vi "ObatainMessage.vi"(8 "error in (no error)":errorcluster, 10 "COM Bluegiga in":refnum<visa-resource-name>, 11 "BLE Message in":refnum<class "BLE Message.lvclass">) -> (0 "error out":errorcluster, 3 "BLE Message out":refnum<class "BLE Message.lvclass">)   [LabVIEW 2015, in "BLE Message.lvclass"]
uses:
  BLE Message.lvclass
  BLE Message.lvclass/BLE Message.ctl
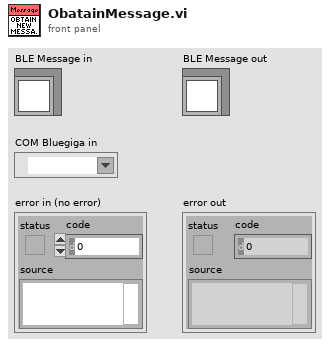
[diagram p1: front panel]
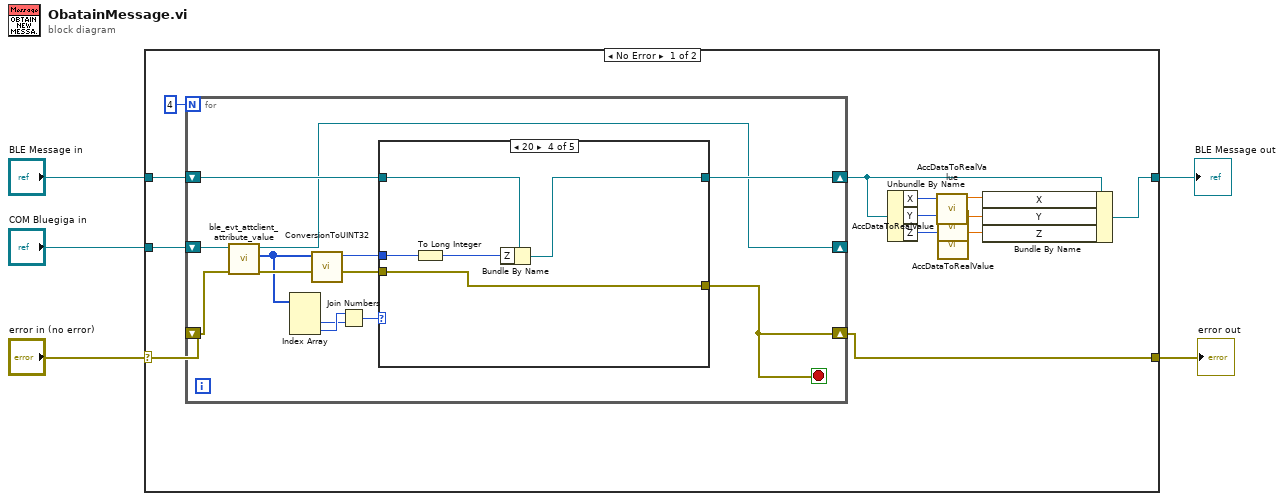
[diagram p0: block diagram]
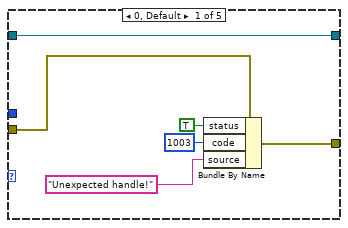
[diagram p2: hidden frame]
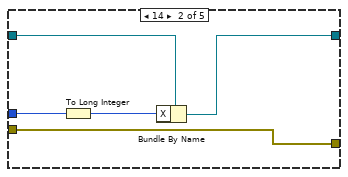
[diagram p3: hidden frame]
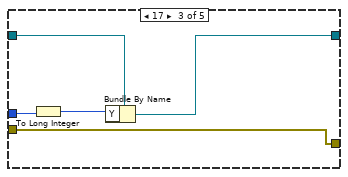
[diagram p4: hidden frame]
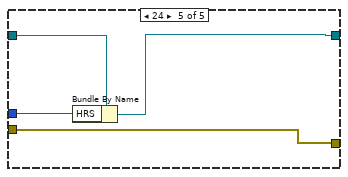
[diagram p5: hidden frame]
diagram:
  n1 = case shown="No Error" "error in (no error)" {
    selector: "error in (no error)" -> [w16 w57]
    tunnel: [w14 w57] -> w4
    tunnel: [w6 w56] -> w2
    tunnel: "BLE Message in" -> [w18 w56]
    tunnel: "COM Bluegiga in" -> [w17 _]
    frame No Error {
      n2 = for {
        N: 4 -> [_]
        shift-right: [w20] -> w14
        shift-left: w16 -> [w29]
        shift-right: [w21] -> w13
        shift-left: w18 -> [w26]
        shift-right: [w19] -> _
        shift-left: w17 -> [w30]
        stop <- w20 stop-if-true
        n3 = call <vilib>:"ble_evt_attclient_attribute_value.vi"("error in (no error)"=w29, "COM Bluegiga in"=w30) -> ("error out"=w24:errorcluster, "characteristic value"=w23:u8[], "COM Bluegiga out"=w19:refnum<visa-resource-name>)  [unwired: 6 in, 1 out]
        n4 = Index Array(array=w23) -> (element #2=w27:u8, element #3=w28:u8)  [unwired: 3 in, 1 out]
        n5 = call "ConversionToUINT32.vi"("uint byte tab"=w23) -> ("Outcome"=w22:u32)  [unwired: 10 in]
        n6 = Join Numbers(hi=w28, lo=w27) -> ((hi.lo)=w25:u16)
        n7 = case shown="20" w25 {
          tunnel: w26 -> [w31 w41 w46 w51 w55]
          tunnel: w24 -> [w36 w39 w44 w49 w52]
          tunnel: [w32 w39 w44 w49 w52] -> w20
          tunnel: w22 -> [_ w38 w43 w48 w54]
          tunnel: [w31 w40 w45 w50 w53] -> w21
          frame 0, Default {
            n8 = Bundle By Name(cluster=w36, "status"=TRUE, "code"=1003, "source"="Unexpected handle!") -> (w32:errorcluster)
          }
          frame 14 {
            n9 = To Long Integer(number=w38) -> (32bit integer=w37:i32)
            n10 = Bundle By Name(cluster=w41, "X"=w37) -> (w40:refnum<class "BLE Message.lvclass">)
          }
          frame 17 {
            n11 = To Long Integer(number=w43) -> (32bit integer=w42:i32)
            n12 = Bundle By Name(cluster=w46, "Y"=w42) -> (w45:refnum<class "BLE Message.lvclass">)
          }
          frame 20 {
            n13 = To Long Integer(number=w48) -> (32bit integer=w47:i32)
            n14 = Bundle By Name(cluster=w51, "Z"=w47) -> (w50:refnum<class "BLE Message.lvclass">)
          }
          frame 24 {
            n15 = Bundle By Name(cluster=w55, "HRS"=w54) -> (w53:refnum<class "BLE Message.lvclass">)
          }
        }
      }
      n16 = Unbundle By Name(w13) -> ("X"=w12:i32, "Y"=w10:i32, "Z"=w8:i32)
      n17 = call "AccDataToRealValue.vi"("Input"=w12) -> ("output"=w11:dbl)  [unwired: 10 in]
      n18 = call "AccDataToRealValue.vi"("Input"=w10) -> ("output"=w9:dbl)  [unwired: 10 in]
      n19 = call "AccDataToRealValue.vi"("Input"=w8) -> ("output"=w7:dbl)  [unwired: 10 in]
      n20 = Bundle By Name(cluster=w13, "X"=w11, "Y"=w9, "Z"=w7) -> (w6:refnum<class "BLE Message.lvclass">)
    }
    frame Error {
    }
  }
  "error out" <- w4
  "BLE Message out" <- w2
